vi "Measured Data (A).vi"(0 "LoadProcedure":refnum<k24>, 5 "ProcedureCommandList":string(combo), 7 "Signal X sel":string(combo), 9 "Signal Y sel":string(combo), 11 "error in (no error)":errorcluster) -> (3 "Value Y":dbl[](array[numeric]), 4 "Signal Names":string[](array[string]), 6 "ProcedureCommandList":string[](array[string]), 8 "Value":dbl, 10 "Value X":dbl[](array[numeric]), 14 "XY Graph":cluster{"Values":dbl[], "Values":dbl[]}(graph), 15 "error out":errorcluster)   [LabVIEW 2011]
doc: "View the measured data from the procedure. The command and the command parameter of the procedure can manually selected (advanced version)."
uses:
  C:/Program Files/Metrohm Autolab/Autolab SDK 1.10/EcoChemie.Autolab.Sdk.dll
  EcoChemie.Autolab.Sdk.dll
  C:/Program Files/Metrohm Autolab/Autolab SDK 1.10/EcoChemie100.dll
  EcoChemie100.dll
panel:
  out "Value 2":dbl
  in  "stop":bool
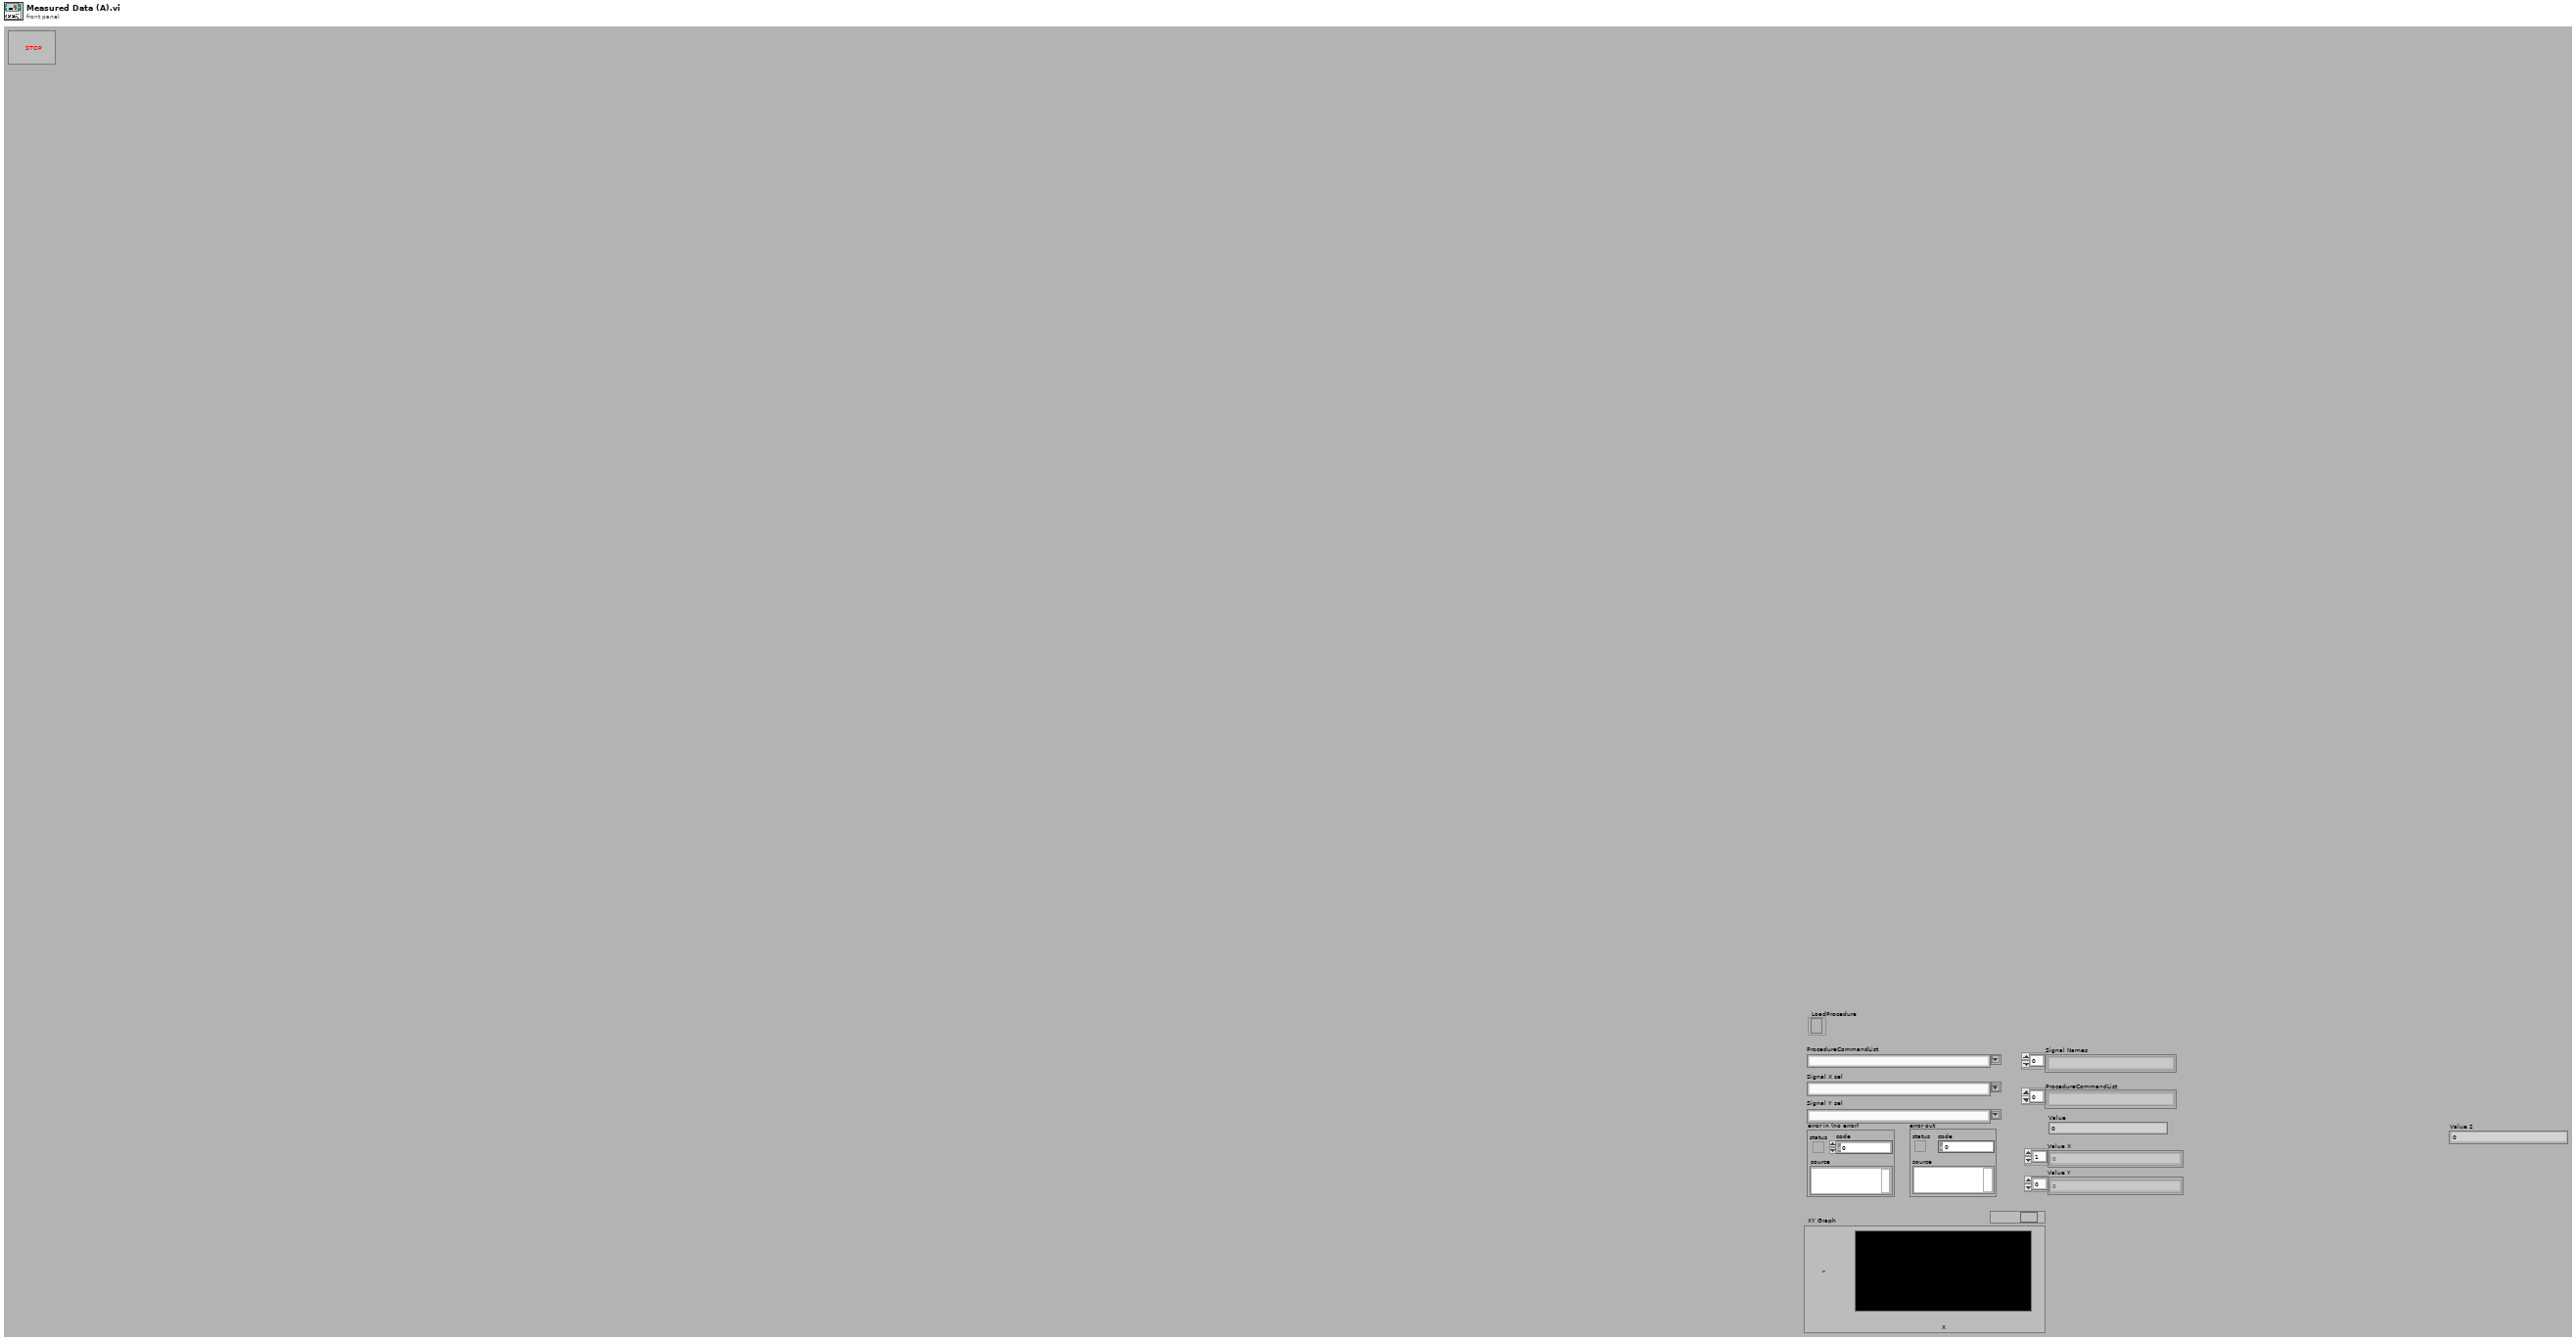
[diagram p1: front panel]
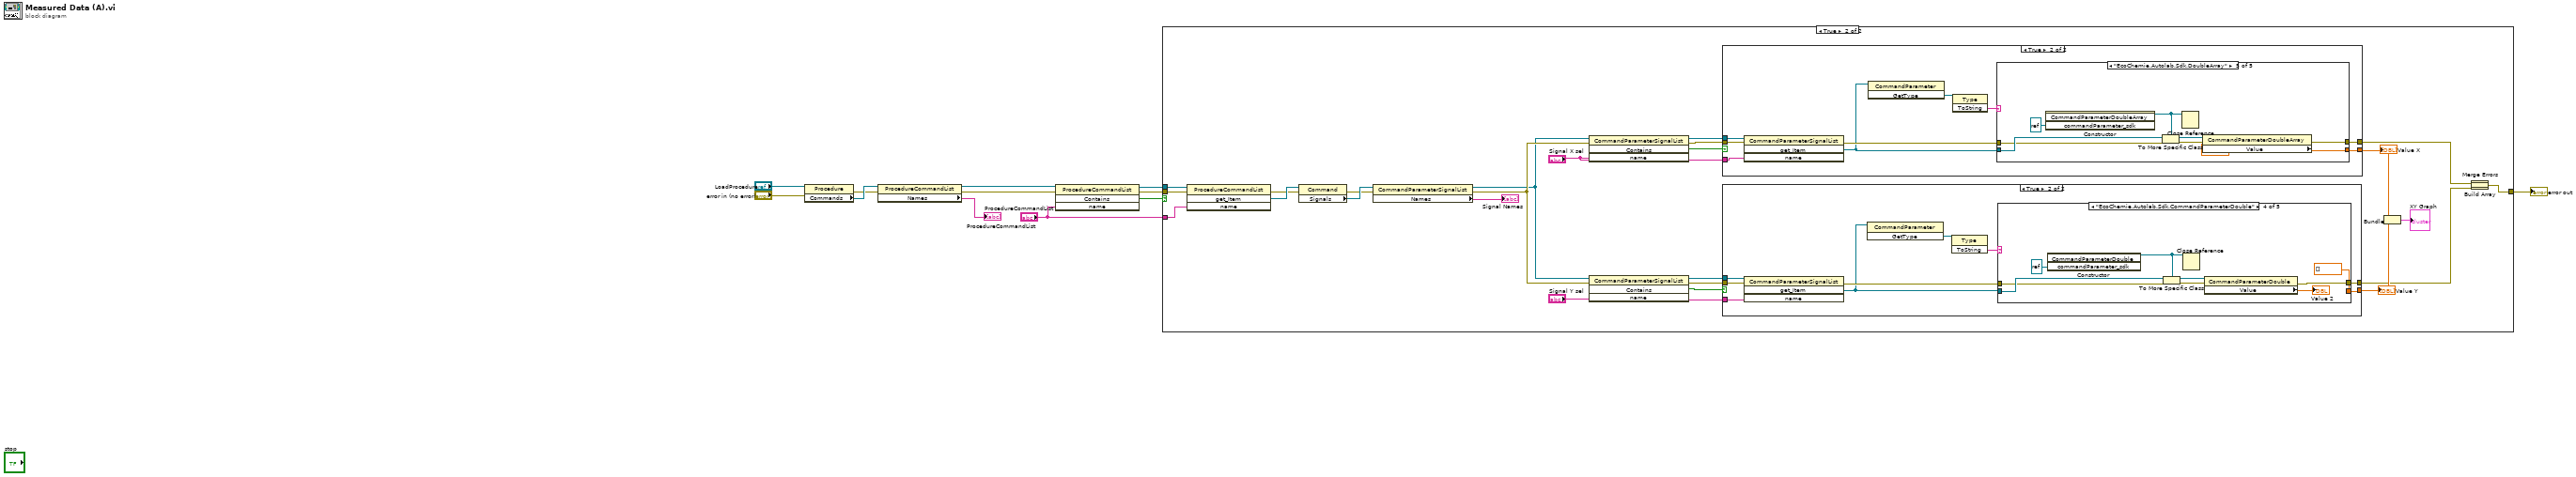
[diagram p0: block diagram]
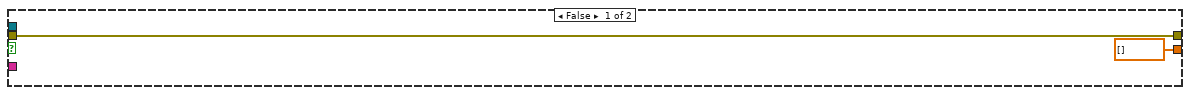
[diagram p3: hidden frame]
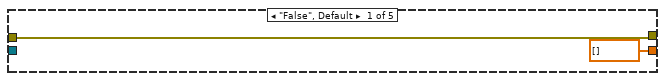
[diagram p4: hidden frame]
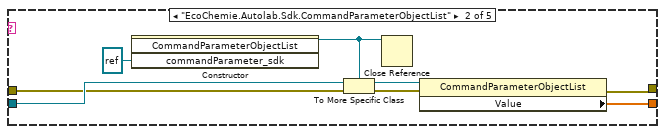
[diagram p5: hidden frame]
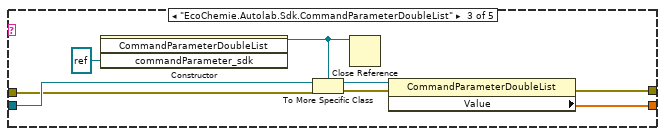
[diagram p6: hidden frame]
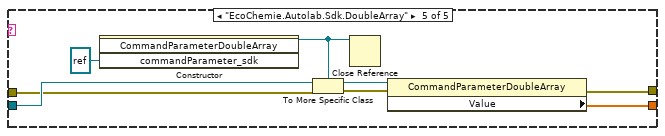
[diagram p7: hidden frame]
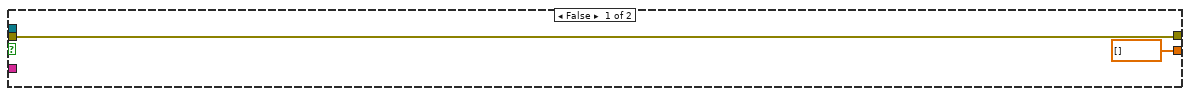
[diagram p8: hidden frame]
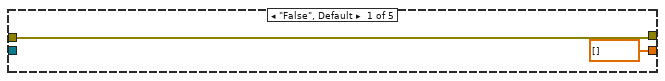
[diagram p9: hidden frame]
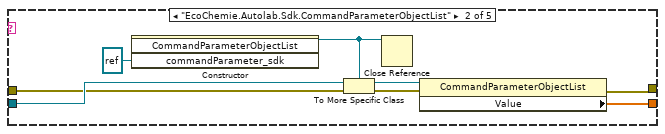
[diagram p10: hidden frame]
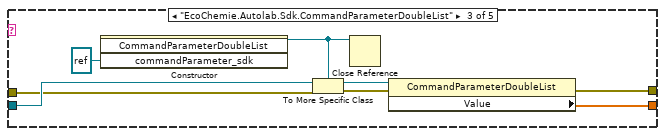
[diagram p11: hidden frame]
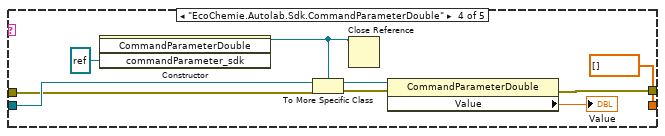
[diagram p12: hidden frame]
diagram:
  n1 = property class="Procedure"(reference="LoadProcedure", error in="error in (no error)") -> (error out=w11:errorcluster, "Commands"=w12:refnum<k24>)  [unwired: 1 out]
  n2 = property class="ProcedureCommandList"(reference=w12, error in=w11) -> (reference out=w10:refnum<k24>, error out=w9:errorcluster, "Names"=→"ProcedureCommandList":string[])
  n3 = invoke class="ProcedureCommandList" method="Contains"(reference=w10, error in=w9, "name"="ProcedureCommandList") -> (reference out=w6:refnum<k24>, error out=w5:errorcluster, "Contains"=w7:bool)  [unwired: 1 in, 1 out]
  n4 = case shown="True" w7 {
    tunnel: "ProcedureCommandList" -> [_ w33]
    tunnel: w6 -> [_ w32]
    tunnel: w5 -> [w13 w31]
    tunnel: [w13 w30] -> w4
    frame False {
    }
    frame True {
      n5 = invoke class="ProcedureCommandList" method="get_Item"(reference=w32, error in=w31, "name"=w33) -> (error out=w37:errorcluster, "get_Item"=w38:refnum<k24>)  [unwired: 1 in, 2 out]
      n6 = property class="Command"(reference=w38, error in=w37) -> (error out=w35:errorcluster, "Signals"=w36:refnum<k24>)  [unwired: 1 out]
      n7 = property class="CommandParameterSignalList"(reference=w36, error in=w35) -> (reference out=w28:refnum<k24>, error out=w29:errorcluster, "Names"=→"Signal Names":string[])
      n8 = invoke class="CommandParameterSignalList" method="Contains"(reference=w28, error in=w29, "name"="Signal X sel") -> (reference out=w24:refnum<k24>, error out=w23:errorcluster, "Contains"=w16:bool)  [unwired: 1 in, 1 out]
      n9 = invoke class="CommandParameterSignalList" method="Contains"(reference=w28, error in=w29, "name"="Signal Y sel") -> (reference out=w22:refnum<k24>, error out=w21:errorcluster, "Contains"=w15:bool)  [unwired: 1 in, 1 out]
      n10 = case shown="True" w15 {
        tunnel: w22 -> [_ w49]
        tunnel: w21 -> [w39 w48]
        tunnel: "Signal Y sel" -> [_ w47]
        tunnel: [dbl[] [] ("ListAsArray") w45] -> w25
        tunnel: [w39 w44] -> w17
        frame False {
        }
        frame True {
          n11 = invoke class="CommandParameterSignalList" method="get_Item"(reference=w49, error in=w48, "name"=w47) -> (error out=w43:errorcluster, "get_Item"=w42:refnum<k24>)  [unwired: 1 in, 2 out]
          n12 = invoke class="CommandParameter" method="GetType"(reference=w42) -> ("GetType"=w46:refnum<k24>)  [unwired: 2 in, 2 out]
          n13 = invoke class="Type" method="ToString"(reference=w46) -> ("ToString"=w41:string)  [unwired: 2 in, 2 out]
          n14 = case shown="\"EcoChemie.Autolab.Sdk.CommandParameterDouble\"" w41 {
            tunnel: w42 -> [_ w56 w65 w74 w82]
            tunnel: w43 -> [w50 w55 w64 w73 w81]
            tunnel: [dbl[] [] ("Value") w57 w63 dbl[] [] ("Value") w80] -> w45
            tunnel: [w50 w54 w62 w71 w79] -> w44
            frame "False", Default {
            }
            frame "EcoChemie.Autolab.Sdk.CommandParameterObjectList" {
              n15 = constructor class="CommandParameterObjectList"("commandParameter_sdk"=refnum<k24> refnum) -> (reference out=w53:refnum<k24>)  [unwired: 3 in, 3 out]
              n16 = To More Specific Class(target class=w53, reference=w56, error in=w55) -> (specific class reference=w59:refnum<k24>, error out=w58:errorcluster)
              n17 = Close Reference(reference=w53) -> ()  [unwired: 1 in, 1 out]
              n18 = property class="CommandParameterObjectList"(reference=w59, error in=w58) -> (error out=w54:errorcluster, "Value"=w57:dbl[])  [unwired: 1 out]
            }
            frame "EcoChemie.Autolab.Sdk.CommandParameterDoubleList" {
              n19 = constructor class="CommandParameterDoubleList"("commandParameter_sdk"=refnum<k24> refnum) -> (reference out=w61:refnum<k24>)  [unwired: 3 in, 3 out]
              n20 = To More Specific Class(target class=w61, reference=w65, error in=w64) -> (specific class reference=w67:refnum<k24>, error out=w66:errorcluster)
              n21 = Close Reference(reference=w61) -> ()  [unwired: 1 in, 1 out]
              n22 = property class="CommandParameterDoubleList"(reference=w67, error in=w66) -> (error out=w62:errorcluster, "Value"=w63:dbl[])  [unwired: 1 out]
            }
            frame "EcoChemie.Autolab.Sdk.CommandParameterDouble" {
              n23 = constructor class="CommandParameterDouble"("commandParameter_sdk"=refnum<k24> refnum) -> (reference out=w69:refnum<k24>)  [unwired: 3 in, 3 out]
              n24 = To More Specific Class(target class=w69, reference=w74, error in=w73) -> (specific class reference=w76:refnum<k24>, error out=w75:errorcluster)
              n25 = Close Reference(reference=w69) -> ()  [unwired: 1 in, 1 out]
              n26 = property class="CommandParameterDouble"(reference=w76, error in=w75) -> (error out=w71:errorcluster, "Value"=→"Value 2":dbl)  [unwired: 1 out]
            }
            frame "EcoChemie.Autolab.Sdk.DoubleArray" {
              n27 = constructor class="CommandParameterDoubleArray"("commandParameter_sdk"=refnum<k24> refnum) -> (reference out=w78:refnum<k24>)  [unwired: 3 in, 3 out]
              n28 = To More Specific Class(target class=w78, reference=w82, error in=w81) -> (specific class reference=w84:refnum<k24>, error out=w83:errorcluster)
              n29 = Close Reference(reference=w78) -> ()  [unwired: 1 in, 1 out]
              n30 = property class="CommandParameterDoubleArray"(reference=w84, error in=w83) -> (error out=w79:errorcluster, "Value"=w80:dbl[])  [unwired: 1 out]
            }
          }
        }
      }
      "Value Y" <- w25
      n31 = case shown="True" w16 {
        tunnel: w24 -> [_ w95]
        tunnel: w23 -> [w85 w94]
        tunnel: "Signal X sel" -> [_ w93]
        tunnel: [dbl[] [] ("ListAsArray") w91] -> w26
        tunnel: [w85 w90] -> w18
        frame False {
        }
        frame True {
          (unwired) dbl[] [] ("ListAsArray")
          n32 = invoke class="CommandParameterSignalList" method="get_Item"(reference=w95, error in=w94, "name"=w93) -> (error out=w92:errorcluster, "get_Item"=w89:refnum<k24>)  [unwired: 1 in, 2 out]
          n33 = invoke class="CommandParameter" method="GetType"(reference=w89) -> ("GetType"=w87:refnum<k24>)  [unwired: 2 in, 2 out]
          n34 = invoke class="Type" method="ToString"(reference=w87) -> ("ToString"=w88:string)  [unwired: 2 in, 2 out]
          n35 = case shown="\"EcoChemie.Autolab.Sdk.DoubleArray\"" w88 {
            tunnel: w89 -> [_ w102 w111 w120 w128]
            tunnel: w92 -> [w96 w101 w110 w119 w127]
            tunnel: [dbl[] [] ("Value") w103 w109 dbl[] [] ("Value") w126] -> w91
            tunnel: [w96 w100 w108 w117 w125] -> w90
            frame "False", Default {
            }
            frame "EcoChemie.Autolab.Sdk.CommandParameterObjectList" {
              n36 = constructor class="CommandParameterObjectList"("commandParameter_sdk"=refnum<k24> refnum) -> (reference out=w99:refnum<k24>)  [unwired: 3 in, 3 out]
              n37 = To More Specific Class(target class=w99, reference=w102, error in=w101) -> (specific class reference=w105:refnum<k24>, error out=w104:errorcluster)
              n38 = Close Reference(reference=w99) -> ()  [unwired: 1 in, 1 out]
              n39 = property class="CommandParameterObjectList"(reference=w105, error in=w104) -> (error out=w100:errorcluster, "Value"=w103:dbl[])  [unwired: 1 out]
            }
            frame "EcoChemie.Autolab.Sdk.CommandParameterDoubleList" {
              n40 = constructor class="CommandParameterDoubleList"("commandParameter_sdk"=refnum<k24> refnum) -> (reference out=w107:refnum<k24>)  [unwired: 3 in, 3 out]
              n41 = To More Specific Class(target class=w107, reference=w111, error in=w110) -> (specific class reference=w113:refnum<k24>, error out=w112:errorcluster)
              n42 = Close Reference(reference=w107) -> ()  [unwired: 1 in, 1 out]
              n43 = property class="CommandParameterDoubleList"(reference=w113, error in=w112) -> (error out=w108:errorcluster, "Value"=w109:dbl[])  [unwired: 1 out]
            }
            frame "EcoChemie.Autolab.Sdk.CommandParameterDouble" {
              n44 = constructor class="CommandParameterDouble"("commandParameter_sdk"=refnum<k24> refnum) -> (reference out=w115:refnum<k24>)  [unwired: 3 in, 3 out]
              n45 = To More Specific Class(target class=w115, reference=w120, error in=w119) -> (specific class reference=w122:refnum<k24>, error out=w121:errorcluster)
              n46 = Close Reference(reference=w115) -> ()  [unwired: 1 in, 1 out]
              n47 = property class="CommandParameterDouble"(reference=w122, error in=w121) -> (error out=w117:errorcluster, "Value"=→"Value":dbl)  [unwired: 1 out]
            }
            frame "EcoChemie.Autolab.Sdk.DoubleArray" {
              n48 = constructor class="CommandParameterDoubleArray"("commandParameter_sdk"=refnum<k24> refnum) -> (reference out=w124:refnum<k24>)  [unwired: 3 in, 3 out]
              n49 = To More Specific Class(target class=w124, reference=w128, error in=w127) -> (specific class reference=w130:refnum<k24>, error out=w129:errorcluster)
              n50 = Close Reference(reference=w124) -> ()  [unwired: 1 in, 1 out]
              n51 = property class="CommandParameterDoubleArray"(reference=w130, error in=w129) -> (error out=w125:errorcluster, "Value"=w126:dbl[])  [unwired: 1 out]
            }
          }
        }
      }
      "Value X" <- w26
      n52 = Bundle("Value"=w26, "Value"=w25) -> (→"XY Graph":cluster{"Value":dbl[], "Value":dbl[]})  [unwired: 1 in]
      n53 = Build Array(w18, w17) -> (w14:errorcluster[])
      n54 = Merge Errors(w14) -> (w30:errorcluster)
    }
  }
  "error out" <- w4
